vi "Keithley2400series_s2x2_ST.vi"() -> ()   [LabVIEW 2014]
uses:
  <vilib>/Utility/file.llb/Write To Spreadsheet File (string).vi
panel:
  in  "Независимое упр.":bool
  in  "+ИП2":bool
  in  "VISA resource name2":refnum<visa-resource-name>
  out "SEEcount 2":dbl
  in  "SEE_th 2":dbl format="%.2f"
  out "Meas 2":dbl format="%#.6g"
  in  "Режим ИП 2  (0: Voltage)":u16(ring) items=["Voltage", "Current"]
  in  "Ограничение ИП2":dbl format="%.2f"
  in  "Выход ИП2":dbl
  out "SEEcount 1":dbl
  in  "SEE_th 1":dbl format="%.2f"
  out "Meas 1":dbl format="%#.6g"
  in  "stop":bool
  in  "Режим ИП1 (0: Voltage)":u16(ring) items=["Voltage", "Current"]
  in  "VISA resource name 1":refnum<visa-resource-name>
  in  "Serial Configuration":T1={"Baud Rate"=9600, "Parity"=0, "Data Bits"=8, "Stop Bits"=10, "Flow Control"=0} {"Flow Control" items=["None", "XON/XOFF", "RTS/CTS", "XON/XOFF & RTS/CTS", "DTR/DSR", "XON/XOFF & DTR/DSR"]; "Stop Bits" items=["1.0"=10, "1.5"=15, "2.0"=20]; "Data Bits" items=["7"=7, "8"=8]; "Parity" items=["None", "Odd", "Even", "Mark", "Space"]; "Baud Rate" items=["300"=300, "600"=600, "1200"=1200, "2400"=2400, "4800"=4800, "9600"=9600, "19200"=19200]}
  in  "Файл записи замеров":path
  in  "Ограничение ИП1":dbl format="%.2f"
  in  "Выход ИП1":dbl
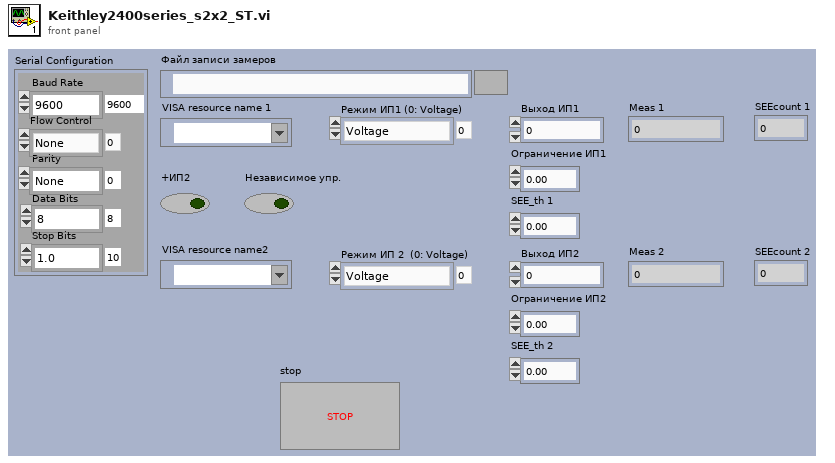
[diagram p1: front panel]
types:
  T1 = cluster{"Baud Rate":u32, "Parity":u16, "Data Bits":u16, "Stop Bits":u16, "Flow Control":u16}
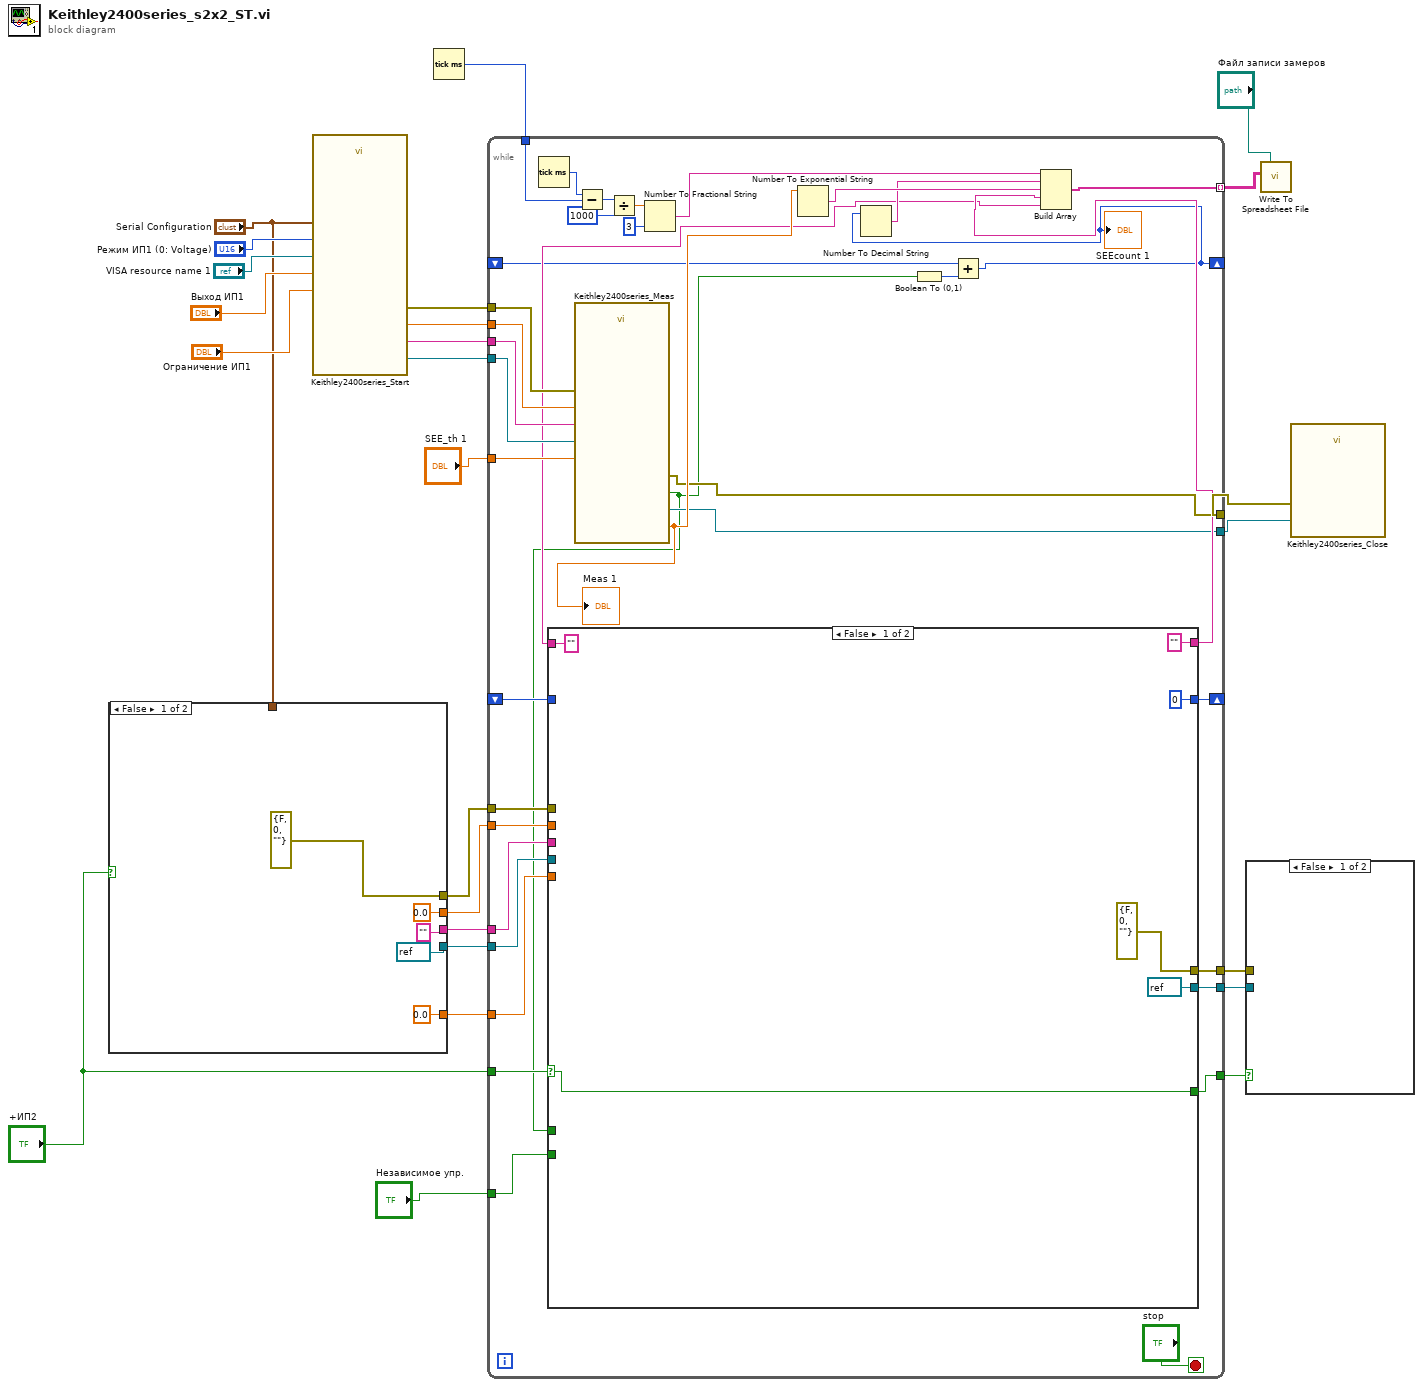
[diagram p0: block diagram]
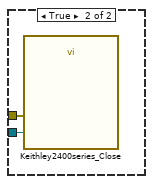
[diagram p2: hidden frame]
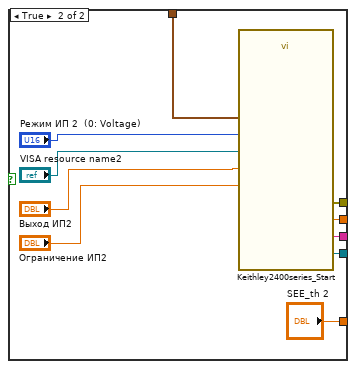
[diagram p3: hidden frame]
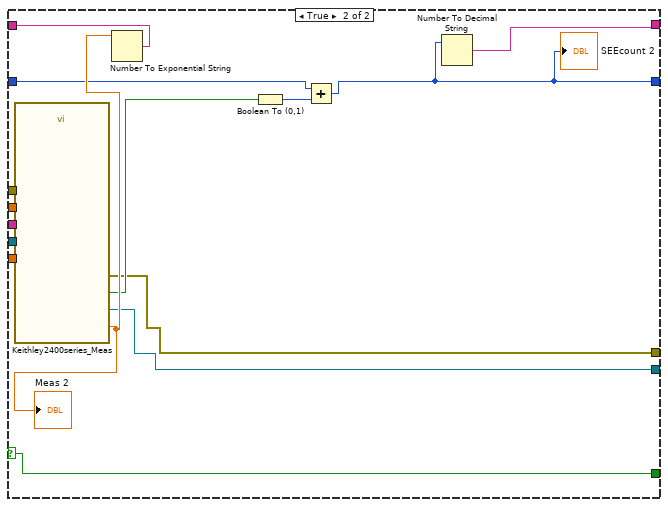
[diagram p4: hidden frame]
diagram:
  n1 = case shown="False" "+ИП2" {
    tunnel: "Serial Configuration" -> [_ w40]
    tunnel: [0.0 ("SEE_th 2") "SEE_th 2"] -> w10
    tunnel: [refnum<visa-resource-name> refnum ("VISA resource name out") w34] -> w9
    tunnel: ["" ("MEAS:Out") w33] -> w8
    tunnel: [0.0 ("MEAS mode 0,Volt") w32] -> w7
    tunnel: [errorcluster {"status"=FALSE, "code"=0, "source"=""} ("error out") w31] -> w6
    frame False {
    }
    frame True {
      n2 = call "Keithley2400series_Start.vi"("Serial Configuration"=w40, "Source Mode  (0: Voltage) 2"="Режим ИП 2  (0: Voltage)", "Ограничение"="Ограничение ИП2", "Выход"="Выход ИП2", "VISA resource name"="VISA resource name2") -> ("error out"=w31:errorcluster, "MEAS:Out"=w33:string, "MEAS mode 0,Volt"=w32:dbl, "VISA resource name out"=w34:refnum<visa-resource-name>)
    }
  }
  n3 = call "Keithley2400series_Start.vi"("Serial Configuration"="Serial Configuration", "Source Mode  (0: Voltage) 2"="Режим ИП1 (0: Voltage)", "Ограничение"="Ограничение ИП1", "Выход"="Выход ИП1", "VISA resource name"="VISA resource name 1") -> ("error out"=w20:errorcluster, "MEAS:Out"=w18:string, "MEAS mode 0,Volt"=w19:dbl, "VISA resource name out"=w17:refnum<visa-resource-name>)
  n4 = Tick Count (ms)() -> (millisecond timer value=w21:u32)
  n5 = while {
    tunnel: w21 -> [w73]
    tunnel: w20 -> [w65]
    tunnel: w19 -> [w66]
    tunnel: w18 -> [w67]
    tunnel: w17 -> [w68]
    tunnel: [w57] -> w16 mode=indexing
    tunnel: "SEE_th 1" -> [w69]
    tunnel: [w43] -> w14
    tunnel: [w42] -> w13
    shift-right: [w47] -> _
    shift-left: _ -> [w48]
    tunnel: w10 -> [w62]
    tunnel: w9 -> [w61]
    tunnel: w8 -> [w60]
    tunnel: w7 -> [w59]
    tunnel: w6 -> [w58]
    shift-right: [w46] -> _
    shift-left: _ -> [w45]
    tunnel: [w54] -> w5
    tunnel: [w53] -> w4
    tunnel: "+ИП2" -> [w52]
    tunnel: [w51] -> w2
    tunnel: "Независимое упр." -> [w50]
    stop <- "stop" stop-if-true
    n6 = Tick Count (ms)() -> (millisecond timer value=w77:u32)
    n7 = call "Keithley2400series_Meas.vi"("MEAS:<f>"=w67, "error in (no error)"=w65, "MEAS mode, 0 Volt"=w66, "ОРЭ_th"=w69, "VISA resource name in"=w68) -> ("error out"=w43:errorcluster, "SEE"=w41:bool, "Замер"=w70:dbl, "VISA out"=w42:refnum<visa-resource-name>)
    "Meas 1" <- w70
    n8 = case shown="False" w52 {
      selector: w52 -> [w79 w90]
      tunnel: w62 -> [_ w98]
      tunnel: w61 -> [_ w97]
      tunnel: w60 -> [_ w96]
      tunnel: w59 -> [_ w95]
      tunnel: w58 -> [_ w94]
      tunnel: ["" w91] -> w56
      tunnel: ["" w92] -> w55
      tunnel: [errorcluster {"status"=FALSE, "code"=0, "source"=""} ("error out") w85] -> w54
      tunnel: [refnum<visa-resource-name> refnum ("VISA resource name out") w84] -> w53
      tunnel: [w79 w90] -> w51
      tunnel: w50 -> [_ _]
      tunnel: w41 -> [_ _]
      tunnel: [i16 0 w86] -> w46
      tunnel: w45 -> [_ w87]
      frame False {
      }
      frame True {
        n9 = call "Keithley2400series_Meas.vi"("MEAS:<f>"=w96, "error in (no error)"=w94, "MEAS mode, 0 Volt"=w95, "ОРЭ_th"=w98, "VISA resource name in"=w97) -> ("error out"=w85:errorcluster, "SEE"=w88:bool, "Замер"=w93:dbl, "VISA out"=w84:refnum<visa-resource-name>)
        "Meas 2" <- w93
        n10 = Number To Exponential String(number=w93) -> (E-format string=w92:string)  [unwired: 3 in]
        n11 = Boolean To (0,1)(Boolean=w88) -> (0, 1=w89:i16)
        n12 = Add(x=w87, y=w89) -> (x+y=w86:i16)
        "SEEcount 2" <- w86
        n13 = Number To Decimal String(number=w86) -> (decimal integer string=w91:string)  [unwired: 1 in]
      }
    }
    n14 = Subtract(x=w77, y=w73) -> (x-y=w76:u32)
    n15 = Divide(x=w76, y=u32 1000) -> (x/y=w74:dbl)
    n16 = Number To Fractional String(number=w74, precision (6)=i16 3) -> (F-format string=w72:string)  [unwired: 2 in]
    n17 = Number To Exponential String(number=w70) -> (E-format string=w64:string)  [unwired: 3 in]
    n18 = Boolean To (0,1)(Boolean=w41) -> (0, 1=w49:i16)
    n19 = Add(x=w48, y=w49) -> (x+y=w47:i16)
    "SEEcount 1" <- w47
    n20 = Number To Decimal String(number=w47) -> (decimal integer string=w63:string)  [unwired: 1 in]
    n21 = Build Array(w72, w63, w64, w56, w55) -> (w57:string[])
  }
  n22 = case shown="False" w2 {
    tunnel: w5 -> [_ w100]
    tunnel: w4 -> [_ w99]
    frame False {
    }
    frame True {
      n23 = call "Keithley2400series_Close.vi"("error in (no error)"=w100, "VISA resource name"=w99) -> ()
    }
  }
  n24 = call-poly <vilib>:"Write To Spreadsheet File.vi"("2D data"=w16, "file path (dialog if empty)"="Файл записи замеров") -> ()  [unwired: 6 in, 1 out]
  n25 = call "Keithley2400series_Close.vi"("error in (no error)"=w14, "VISA resource name"=w13) -> ()
